vi "GenerateNameplateInfoForAG.vi"(11 "motor nameplate information":T1) -> (1 "stator resistance":dbl[](array[numeric]), 2 "nameplate information for AG":T2, 3 "invalid stator resistance":bool)   [LabVIEW 2017, in "McsaAnalysisFunctions.lvlib"]
doc: "Regenerates the namplate information for Speed Estimation VI and Torque Load and Efficiency VI and estimates the stator resistance values for air gap torque method based on motor nameplate information."
uses:
  <vilib>/addons/InsightCM/Utilities/Analysis/MCSA/McsaAnalysisFunctions.lvlib
  <vilib>/addons/InsightCM/Utilities/Analysis/MCSA/controls/McsaMotor.ctl
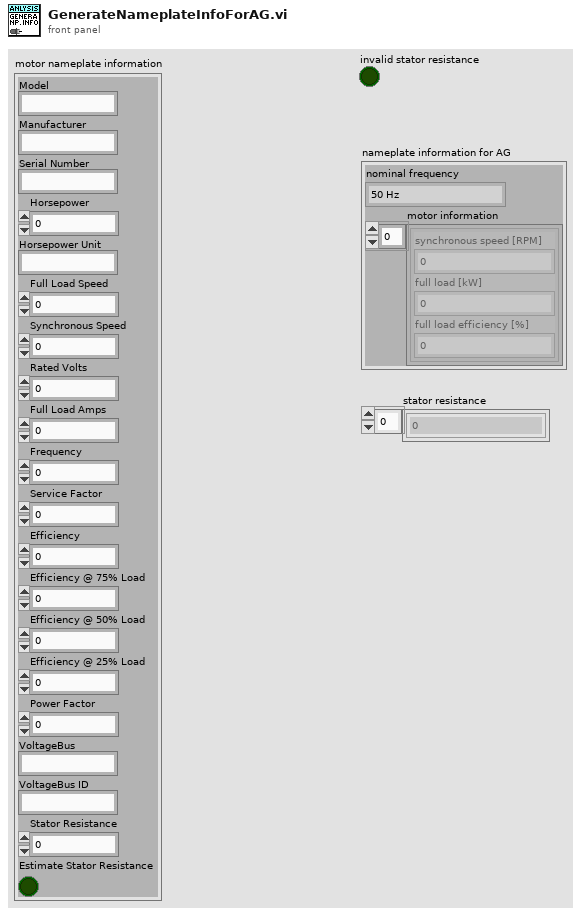
[diagram p1: front panel]
types:
  T1 = typedef "McsaAnalysisFunctions.lvlib/McsaMotor.ctl" = cluster{"Model":string, "Manufacturer":string, "Serial Number":string, "Horsepower":dbl, "Horsepower Unit":string, "Full Load Speed":dbl, "Synchronous Speed":dbl, "Rated Volts":dbl, "Full Load Amps":dbl, "Frequency":dbl, "Service Factor":dbl, "Efficiency":dbl, "Efficiency @ 75% Load":dbl, "Efficiency @ 50% Load":dbl, "Efficiency @ 25% Load":dbl, "Power Factor":dbl, "VoltageBus":string, "VoltageBus ID":string, "Stator Resistance":dbl, "Estimate Stator Resistance":bool}
  T2 = cluster{"nominal frequency":enum16{"50 Hz", "60 Hz"}, "motor information":cluster{"synchronous speed [RPM]":dbl, "full load [kW]":dbl, "full load efficiency [%]":dbl}[]}
  T3 = cluster{"synchronous speed [RPM]":dbl, "full load [kW]":dbl, "full load efficiency [%]":dbl}
  T4 = cluster{"nominal frequency":enum16{"50 Hz", "60 Hz"}, "motor information":cluster{"synchronous speed [RPM]":dbl, "full load [W]":dbl, "full load efficiency [%]":dbl}[]}
  T5 = cluster{"synchronous speed [RPM]":dbl, "full load [kW]":dbl, "full load efficiency [%]":dbl}[]
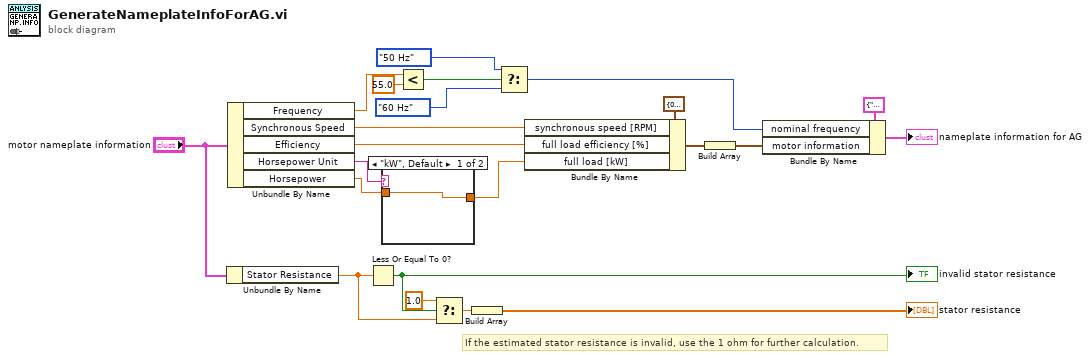
[diagram p0: block diagram]
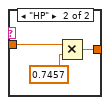
[diagram p2: hidden frame]
diagram:
  # "If the estimated stator resistance is invalid, use the 1 ohm for further calculation."
  n1 = Unbundle By Name("motor nameplate information") -> ("Stator Resistance"=w2:dbl)
  n2 = Unbundle By Name("motor nameplate information") -> ("Frequency"=w15:dbl, "Synchronous Speed"=w18:dbl, "Efficiency"=w7:dbl, "Horsepower Unit"=w10:string, "Horsepower"=w9:dbl)
  n3 = Less Or Equal To 0?(x=w2) -> (x <= 0?=w3:bool)
  "invalid stator resistance" <- w3
  n4 = case shown="\"kW\", Default" w10 {
    tunnel: [w23 w25] -> w6
    tunnel: w9 -> [w23 w26]
    frame "kW", Default {
    }
    frame "HP" {
      n5 = Multiply(x=w26, y=0.7457) -> (x*y=w25:dbl)
    }
  }
  n6 = Less?(x=w15, y=55.0) -> (x < y?=w16:bool)
  n7 = Select(t=1.0, s=w3, f=w2) -> (s? t:f=w4:dbl)
  n8 = Build Array(w4) -> (→"stator resistance":dbl[])
  n9 = Select(t=enum16{"50 Hz", "60 Hz"}."50 Hz" ("nominal frequency"), s=w16, f=enum16{"50 Hz", "60 Hz"}."60 Hz" ("nominal frequency")) -> (s? t:f=w12:enum16{"50 Hz", "60 Hz"})
  n10 = Bundle By Name(cluster=T3 {"synchronous speed [RPM]"=0.0, "full load [kW]"=0.0, "full load efficiency [%]"=0.0} ("motor information"), "synchronous speed [RPM]"=w18, "full load efficiency [%]"=w7, "full load [kW]"=w6) -> (w17:T3)
  n11 = Build Array(w17) -> (w20:T5)
  n12 = Bundle By Name(cluster=T4 {"nominal frequency"=enum."50 Hz", "motor information"=[]} ("nameplate information"), "nominal frequency"=w12, "motor information"=w20) -> (→"nameplate information for AG":T4)
